vi "BC Major Frame End.vi"(8 "error in (no error)":errorcluster, 11 "Bus Controller in":refnum<class "Bus Controller.lvclass">) -> (0 "error out":errorcluster, 3 "Bus Controller out":refnum<class "Bus Controller.lvclass">)   [LabVIEW 2020, in "Unit Tests.lvlib" / "Bus Controller.lvclass"]
uses:
  Bus Controller.lvclass
  Bus Controller.lvclass/Bus Controller.ctl
  Frames & Messages/TypeDefs/BC Op Codes - Verbose.ctl
  Frames & Messages/TypeDefs/BC Condition Codes.ctl
  <vilib>/addons/_JKI Toolkits/Caraya/classes/Assert/Assert True.vi
  Dependencies/FPGA Interface/FPGA Interface.lvclass
  BCI-1553 API.lvlib
  <vilib>/addons/_JKI Toolkits/Caraya/classes/Assert/Assert.lvclass
  <vilib>/addons/_JKI Toolkits/Caraya/classes/Test/Test.lvclass
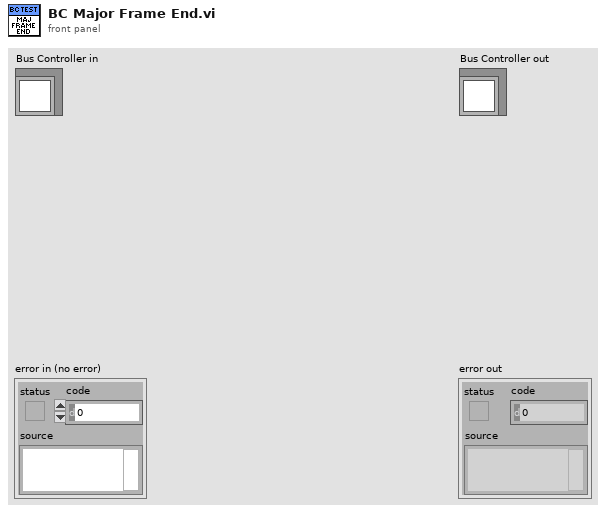
[diagram p1: front panel]
types:
  T1 = typedef "BCI-1553 API.lvlib/BC Condition Codes.ctl" = enum16{"GP0 == 1 || LT", "GP1 == 1 || NE", "GP2 == 1", "GP3 == 1", "GP4 == 1", "GP5 == 1", "GP6 == 1", "GP7 == 1", "NORESP", "FMTERR", "GOODBLOCK", "MSKSTATSET", "BADMSG", "1RETRY", "2RETRY", "ALWAYS"}
  T2 = typedef "BCI-1553 API.lvlib/BC Op Codes - Verbose.ctl" = enum16{"EXECUTE MSG", "EXECUTE MSG GO", "JUMP", "CALL SUBROUTINE", "RETURN", "INTERRUPT REQUEST", "HALT", "DELAY", "WAIT FRAME TIMER = 0", "COMPARE FRAME TIMER", "COMPARE MSG TIMER", "LOAD TIME TAG CTR", "LOAD TIME TAG CTR HI", "LOAD FRAME TIMER", "START FRAME TIMER", "PUSH TIME TAG COUNT", "PUSH TIME TAG COUNT HI", "PUSH TIME TAG COUNT BOTH", "PUSH BLOCK STATUS WORD", "PUSH CURRENT VALUE", "PUSH INDIRECT", "WAIT EXT TRIGGER", "EXECUTE AND FLIP", "EXECUTE, FLIP, GO", "WRITE VALUE TO WMI", "WRITE VALUE TO MEM", "DECREMENT RAM, SKIP", "FLAG"}
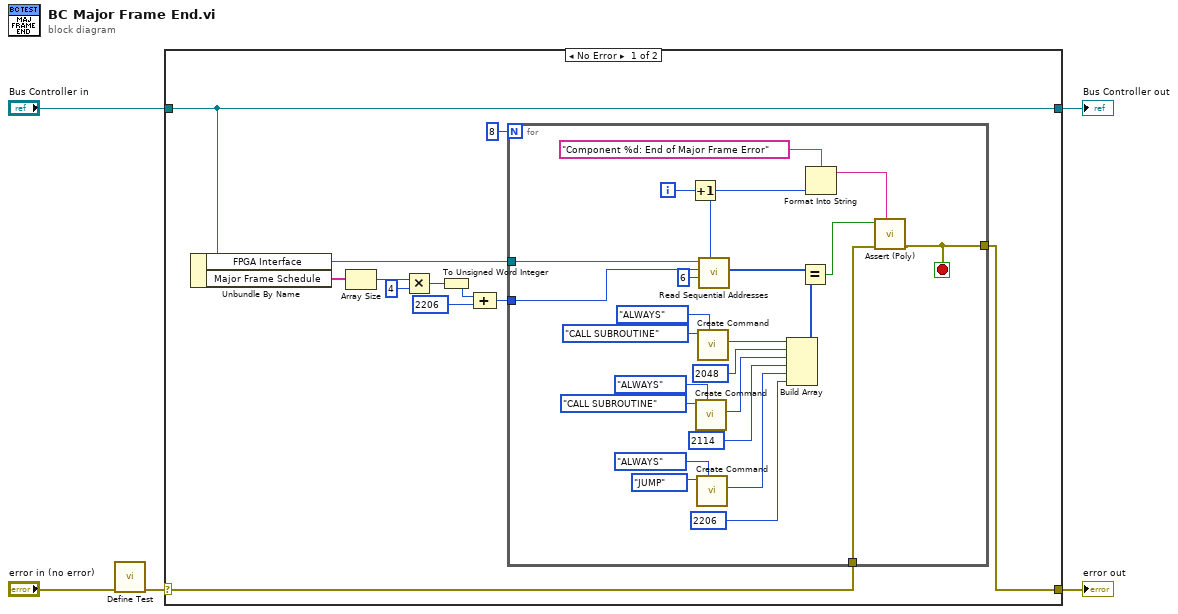
[diagram p0: block diagram]
diagram:
  n1 = call <vilib>:"Define Test.vi"("error in (no error)"="error in (no error)") -> ("error out"=w1:errorcluster)  [unwired: 9 in, 1 out]
  n2 = case shown="No Error" w1 {
    selector: w1 -> [w9 w43]
    tunnel: [w8 w43] -> w5
    tunnel: [w16 w42] -> w3
    tunnel: "Bus Controller in" -> [w16 w42]
    frame No Error {
      n3 = Unbundle By Name(w16) -> ("FPGA Interface"=w15:refnum<class "FPGA Interface.lvclass">, "Major Frame Schedule"=w10:string[])
      n4 = Array Size(array=w10) -> (size(s)=w11:i32)
      n5 = Multiply(x=w11, y=4) -> (x*y=w13:i32)
      n6 = To Unsigned Word Integer(number=w13) -> (unsigned 16bit integer=w14:u16)
      n7 = Compound Arithmetic op=ADD(w14, u16 2206) -> (w7:u16)
      n8 = for {
        N: 8 -> [_]
        tunnel: w15 -> [w41]
        tunnel: w7 -> [w38]
        tunnel: [w26] -> w8
        tunnel: w9 -> [w23]
        i -> [w39]
        stop <- w26 stop-if-true
        n9 = Increment(x=w39) -> (x+1=w36:i32)
        n10 = call "Create Command.vi"("Condition"=BC_Condition_Codes."ALWAYS", "Op Code"=BC_Op_Codes_-_Verbose."CALL SUBROUTINE") -> ("Instruction"=w30:u16)  [unwired: 8 in, 1 out]
        n11 = call "Create Command.vi"("Condition"=BC_Condition_Codes."ALWAYS", "Op Code"=BC_Op_Codes_-_Verbose."JUMP") -> ("Instruction"=w19:u16)  [unwired: 8 in, 1 out]
        n12 = call "Create Command.vi"("Condition"=BC_Condition_Codes."ALWAYS", "Op Code"=BC_Op_Codes_-_Verbose."CALL SUBROUTINE") -> ("Instruction"=w31:u16)  [unwired: 8 in, 1 out]
        n13 = call-dynamic "Read Sequential Addresses.vi"("Target IC (1-8)"=w36, "Addresses to Read"=u16 6, "Starting Address"=w38, "FPGA Interface in"=w41) -> ("Data"=w28:u16[])  [unwired: 6 in, 1 out]
        n14 = Build Array(w31, u16 2048, w30, u16 2114, w19, u16 2206) -> (w29:u16[])
        n15 = Equal?(x=w28, y=w29) -> (x = y?=w24:bool)
        n16 = Format Into String(format string="Component %d: End of Major Frame Error" ("custom report message (\"\")"), w36) -> (resulting string=w25:string)  [unwired: 2 in, 1 out]
        n17 = call-poly <vilib>:"Assert (Poly).vi"("Label"=w25, "error in (no error)"=w23, "True?"=w24) -> ("error out"=w26:errorcluster)  [unwired: 7 in, 1 out]
      }
    }
    frame Error {
    }
  }
  "error out" <- w5
  "Bus Controller out" <- w3
